vi "As PropertyObject.vi"(8 "error in (no error)":errorcluster, 11 "Sequence in":refnum<class "Sequence.lvclass">) -> (0 "error out":errorcluster, 2 "PropertyObject":refnum<k7>, 3 "Sequence out":refnum<class "Sequence.lvclass">)   [LabVIEW 2020, in "TSnax.lvlib" / "Sequence.lvclass"]
uses:
  Sequence.lvclass
  Sequence.lvclass/Sequence.ctl
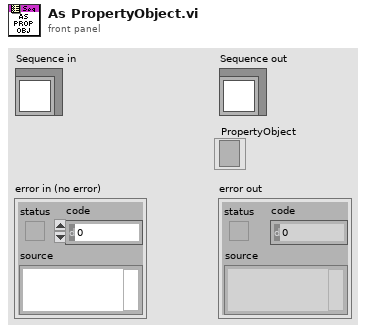
[diagram p1: front panel]
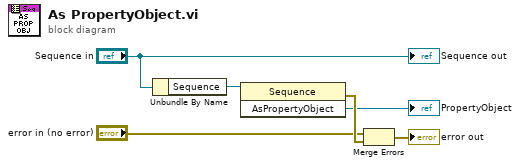
[diagram p0: block diagram]
diagram:
  n1 = Unbundle By Name("Sequence in") -> ("Sequence"=w3:refnum<k7>)
  n2 = invoke class="Sequence" method="AsPropertyObject"(reference=w3) -> (error out=w6:errorcluster, "AsPropertyObject"=→"PropertyObject":refnum<k7>)  [unwired: 2 in, 1 out]
  n3 = Merge Errors("error in (no error)", w6) -> (→"error out":errorcluster)
  "Sequence out" <- "Sequence in"
